vi "Calculatrice.vi"() -> ()   [LabVIEW 2020]
doc: "Calculatrice II - ceci est un programme de calculatrice"
panel:
  out "Local":string
  in  "entrée d'erreur (pas d'erreur)":errorcluster
  in  "Btn_Error":bool caption="Error"
  out "sortie d'erreur":errorcluster
  in  "Btn_Stop":bool
  out "Display":cluster{"Num":dbl, "Char":string}
  in  "Pad":T1
  # "Calculatrice"
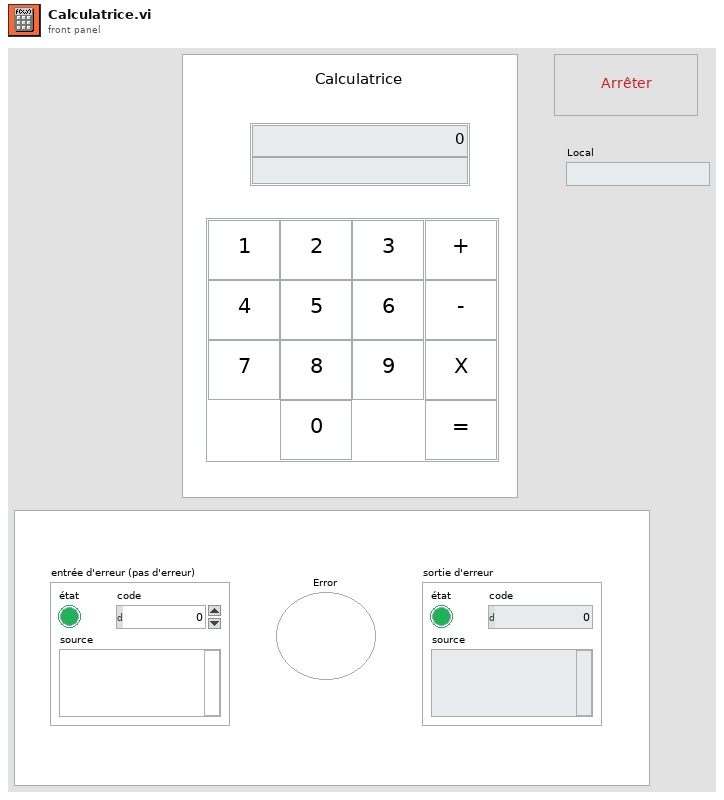
[diagram p1: front panel]
types:
  T1 = cluster{"Btn_1":bool, "Btn_2":bool, "Btn_3":bool, "Btn_4":bool, "Btn_5":bool, "Btn_6":bool, "Btn_7":bool, "Btn_8":bool, "Btn_9":bool, "Btn_0":bool, "Btn_+":bool, "Btn_-":bool, "Btn_X":bool, "Btn_=":bool}
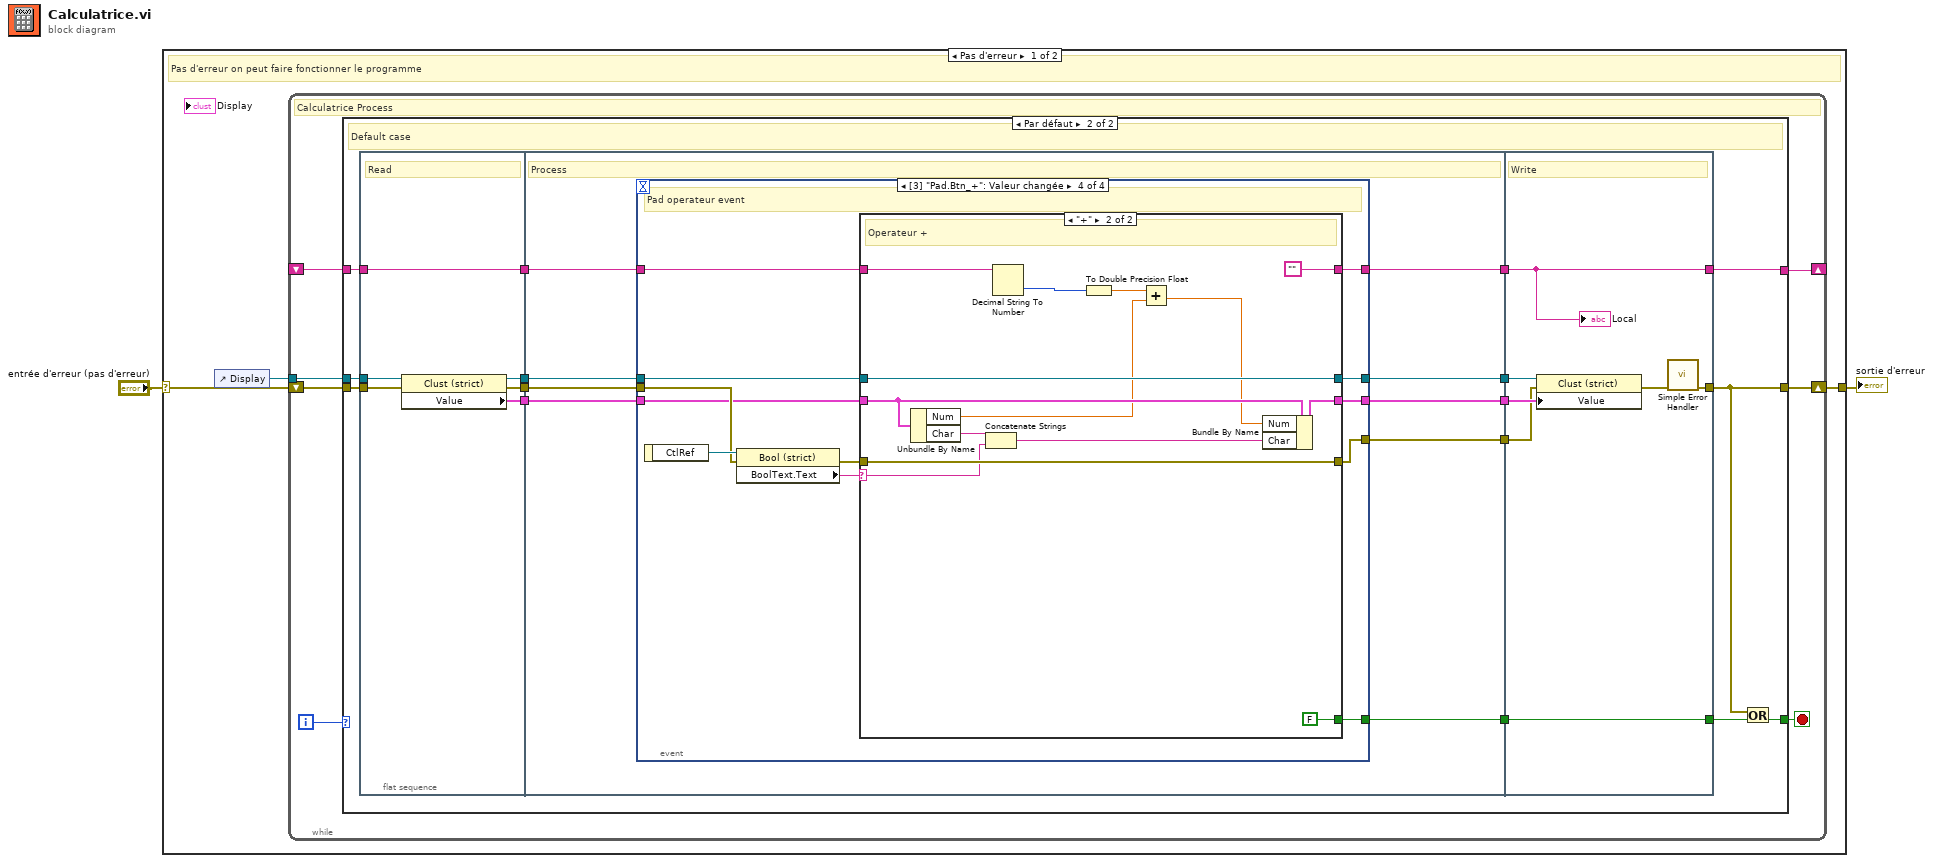
[diagram p0: block diagram]
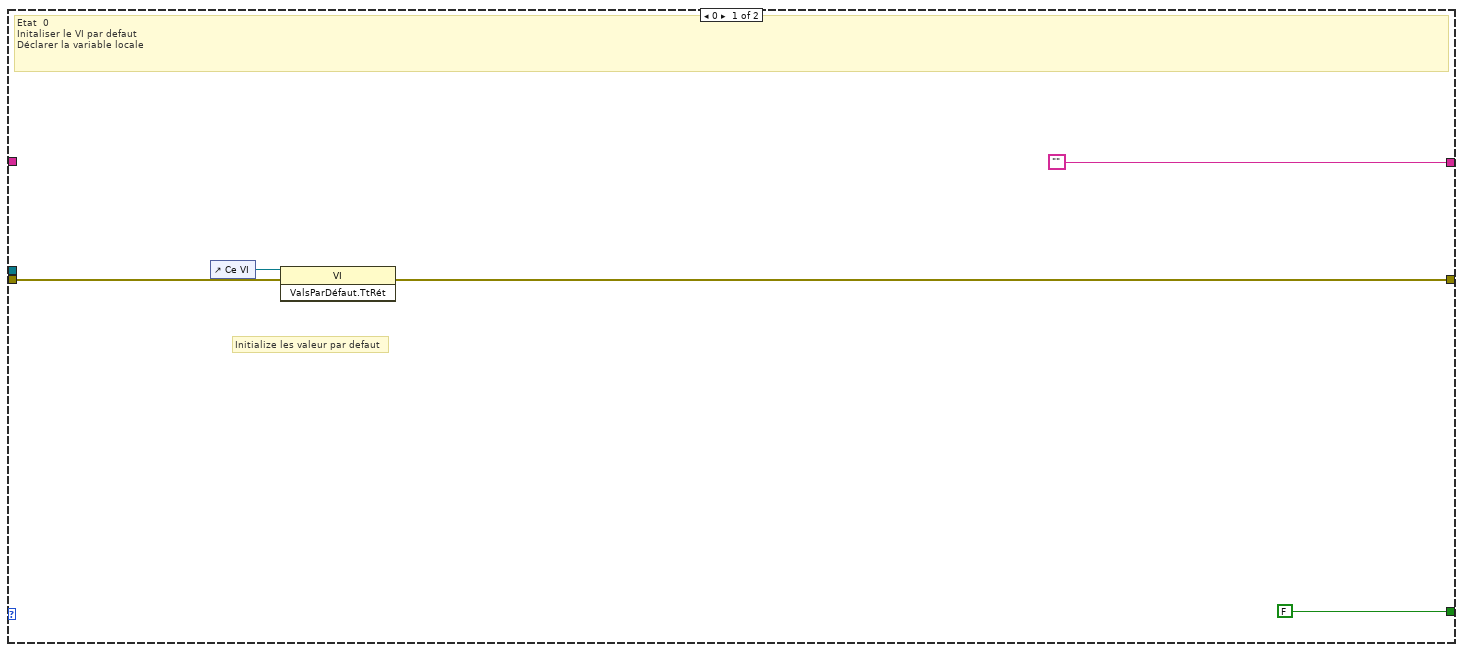
[diagram p2: hidden frame]
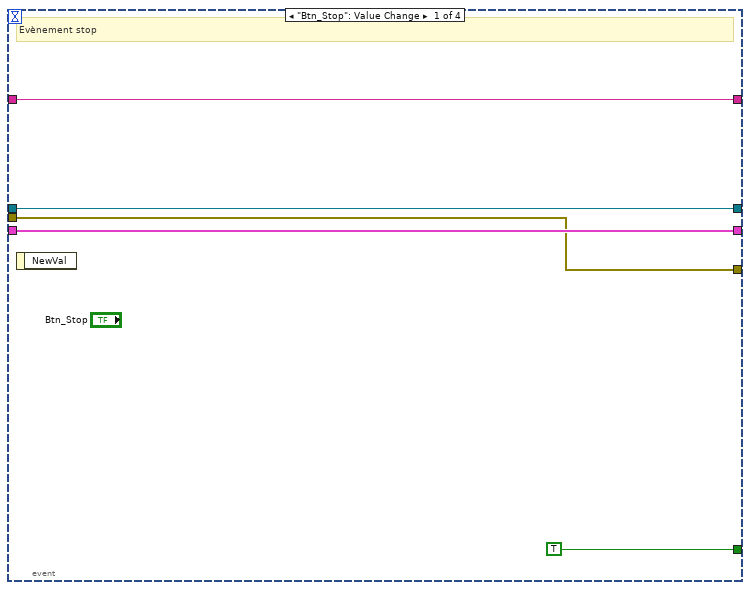
[diagram p3: hidden frame]
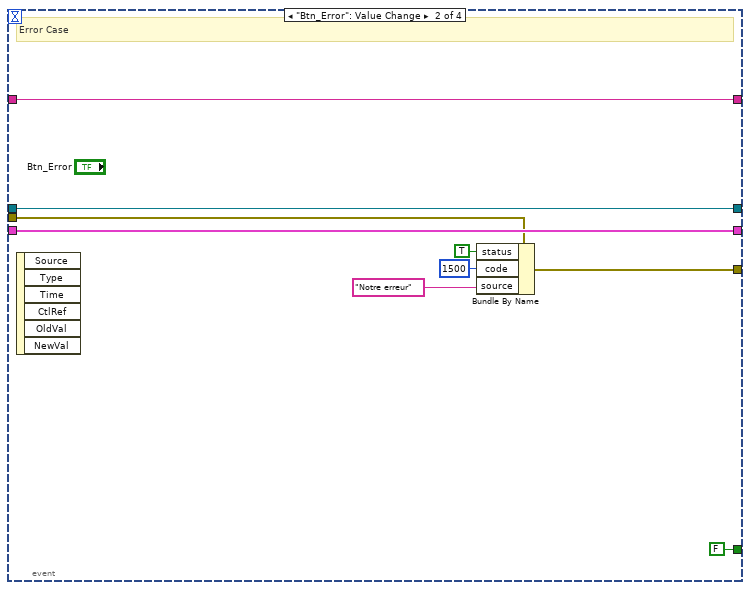
[diagram p4: hidden frame]
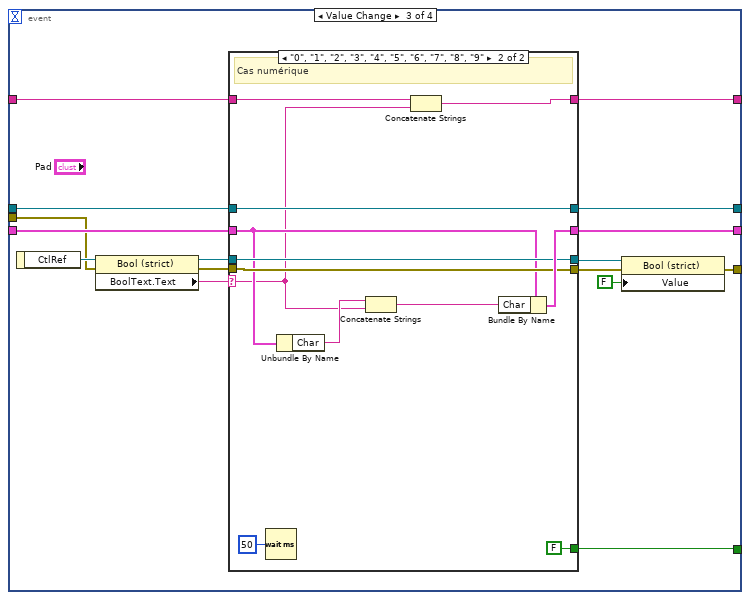
[diagram p5: hidden frame]
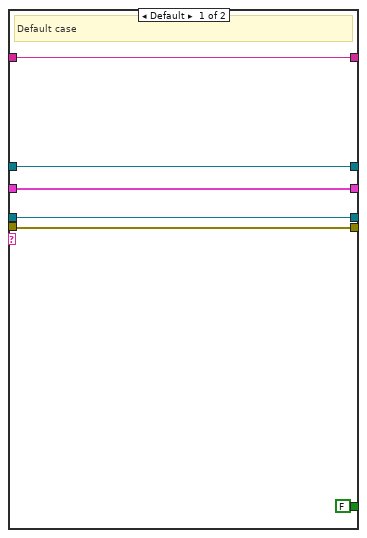
[diagram p6: hidden frame]
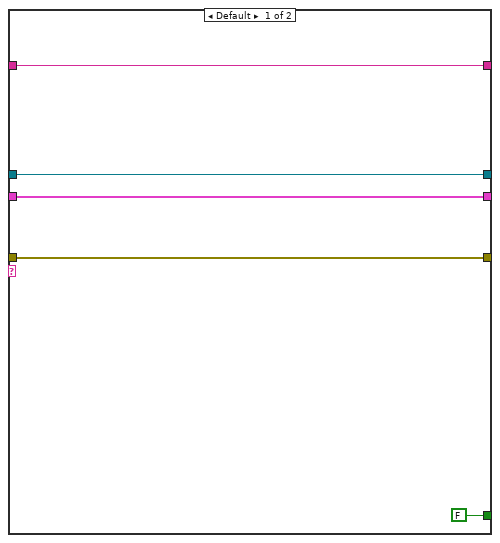
[diagram p7: hidden frame]
diagram:
  n1 = case shown="Pas d'erreur" "entrée d'erreur (pas d'erreur)" {
    selector: "entrée d'erreur (pas d'erreur)" -> [w3 w135]
    tunnel: [w4 w135] -> w2
    frame No Error {
      # "Pas d'erreur on peut faire fonctionner le programme"
      n2 = control-ref of="Display"() -> (w5:refnum<vi>)
      n3 = while {
        tunnel: w5 -> [w12]
        shift-right: [w10] -> w4
        shift-left: w3 -> [w8]
        shift-right: [w7] -> _
        shift-left: _ -> [w6]
        i -> [w9]
        stop <- w11 stop-if-true
        # "Calculatrice Process"
        n4 = case shown="Par défaut" w9 {
          tunnel: w12 -> [_ w25]
          tunnel: w8 -> [w15 w24]
          tunnel: [FALSE w23] -> w11
          tunnel: [w14 w22] -> w10
          tunnel: ["" w18] -> w7
          tunnel: w6 -> [_ w21]
          frame 0 {
            # "Initialize les valeur par defaut"
            # "Etat  0\nInitaliser le VI par defaut\nDéclarer la variable locale"
            n5 = control-ref of="Ce VI"() -> (w16:refnum<vi>)
            n6 = invoke class="VI" method="ValsParDéfaut.TtRét"(reference=w16, error in=w15) -> (error out=w14:errorcluster)  [unwired: 1 in, 2 out]
          }
          frame Default {
            # "Default case"
            n7 = flat-sequence {
              tunnel: w25 -> [w39]
              tunnel: [w38] -> w33
              tunnel: [w37] -> w32
              tunnel: w24 -> [w35]
              tunnel: [w36] -> w31
              tunnel: w21 -> [w34]
              tunnel: [w34] -> w20
              tunnel: [w48] -> w30
              tunnel: w33 -> [w47]
              tunnel: w32 -> [w46]
              tunnel: [w45] -> w29
              tunnel: [w44] -> w28
              tunnel: w31 -> [w43]
              tunnel: [w42] -> w27
              tunnel: w20 -> [w41]
              tunnel: [w40] -> w19
              tunnel: [w134] -> w26
              tunnel: w30 -> [w134]
              tunnel: w29 -> [w133]
              tunnel: w28 -> [w132]
              tunnel: w27 -> [w131]
              tunnel: [w129] -> w22
              tunnel: w19 -> [w128]
              tunnel: [w128] -> w18
              frame #0 {
                # "Read"
                n8 = property class="Clust (strict)"(reference=w39, error in=w35) -> (reference out=w37:refnum<vi>, error out=w36:errorcluster, "Value"=w38:cluster{"Num":dbl, "Char":string})
              }
              frame #1 {
                # "Process"
                n9 = event shown="[3] \"Pad.Btn_+\": Valeur changée" {
                  selector: _ -> [_ _ _ _]
                  dyn-events: _ -> [_ _ _ _]
                  timeout: _ -> [_ _ _ _]
                  tunnel: [TRUE FALSE w76 w108] -> w48
                  tunnel: w47 -> [w51 w60 w75 w104]
                  tunnel: w46 -> [w52 w61 w74 w105]
                  tunnel: [w52 w61 w73 w102] -> w45
                  tunnel: [w51 w60 w72 w103] -> w44
                  tunnel: w43 -> [w50 w59 w68 w106]
                  tunnel: [w50 w58 w65 w99] -> w42
                  tunnel: w41 -> [w49 w54 w64 w98]
                  tunnel: [w49 w54 w63 w97] -> w40
                  event "Btn_Stop": Value Change {
                    # "Evènement stop"
                    n10 = event-data() -> ()  [unwired: 1 in, 1 out]
                  }
                  event "Btn_Error": Value Change {
                    # "Error Case"
                    n11 = event-data() -> ()  [unwired: 1 in, 6 out]
                    n12 = Bundle By Name(cluster=w59, "status"=TRUE, "code"=1500, "source"="Notre erreur") -> (w58:errorcluster)
                  }
                  event "Pad.Btn_1", "Pad.Btn_2", "Pad.Btn_3", "Pad.Btn_4", "Pad.Btn_5", "Pad.Btn_6", "Pad.Btn_7", "Pad.Btn_8", "Pad.Btn_9", "Pad.Btn_0": Value Change {
                    n13 = event-data() -> ("CtlRef"=w78:refnum<vi>)  [unwired: 1 in]
                    n14 = property class="Bool (strict)"(reference=w78, error in=w68) -> (reference out=w71:refnum<vi>, error out=w67:errorcluster, "BoolText.Text"=w77:string)
                    n15 = case shown="\"0\", \"1\", \"2\", \"3\", \"4\", \"5\", \"6\", \"7\", \"8\", \"9\"" w77 {
                      selector: w77 -> [_ w85]
                      tunnel: [FALSE FALSE] -> w76
                      tunnel: w75 -> [w82 w90]
                      tunnel: w74 -> [w83 w95]
                      tunnel: [w83 w95] -> w73
                      tunnel: [w82 w94] -> w72
                      tunnel: w71 -> [w81 w93]
                      tunnel: [w81 w93] -> w70
                      tunnel: w67 -> [w80 w91]
                      tunnel: [w80 w91] -> w66
                      tunnel: w64 -> [w79 w88]
                      tunnel: [w79 w86] -> w63
                      frame Default {
                        # "Default case"
                      }
                      frame "0", "1", "2", "3", "4", "5", "6", "7", "8", "9" {
                        # "Cas numérique"
                        n16 = Wait (ms)(milliseconds to wait=u32 50 ("attente (ms)")) -> ()  [unwired: 1 out]
                        n17 = Unbundle By Name(w90) -> ("Char"=w89:string)
                        n18 = Concatenate Strings(w89, w85) -> (w87:string)
                        n19 = Concatenate Strings(w88, w85) -> (w86:string)
                        n20 = Bundle By Name(cluster=w90, "Char"=w87) -> (w94:cluster{"Num":dbl, "Char":string})
                      }
                    }
                    n21 = property class="Bool (strict)"(reference=w70, error in=w66, "Value"=FALSE ("Valeur")) -> (error out=w65:errorcluster)  [unwired: 1 out]
                  }
                  event "Pad.Btn_+": Value Change {
                    # "Pad operateur event"
                    n22 = event-data() -> ("CtlRef"=w107:refnum<vi>)  [unwired: 1 in]
                    n23 = property class="Bool (strict)"(reference=w107, error in=w106) -> (error out=w100:errorcluster, "BoolText.Text"=w101:string)  [unwired: 1 out]
                    n24 = case shown="\"+\"" w101 {
                      selector: w101 -> [_ w121]
                      tunnel: [FALSE FALSE] -> w108
                      tunnel: w105 -> [w111 w126]
                      tunnel: w104 -> [w112 w123]
                      tunnel: [w112 w124] -> w103
                      tunnel: [w111 w126] -> w102
                      tunnel: w100 -> [w110 w125]
                      tunnel: [w110 w125] -> w99
                      tunnel: w98 -> [w109 w118]
                      tunnel: [w109 ""] -> w97
                      frame Default {
                      }
                      frame "+" {
                        # "Operateur +"
                        n25 = Unbundle By Name(w123) -> ("Num"=w114:dbl, "Char"=w122:string)
                        n26 = Concatenate Strings(w122, w121) -> (w120:string)
                        n27 = Decimal String To Number(string=w118) -> (number=w117:i32)  [unwired: 2 in, 1 out]
                        n28 = To Double Precision Float(number=w117) -> (double precision float=w116:dbl)
                        n29 = Add(x=w116, y=w114) -> (x+y=w115:dbl)
                        n30 = Bundle By Name(cluster=w123, "Num"=w115, "Char"=w120) -> (w124:cluster{"Num":dbl, "Char":string})
                      }
                    }
                  }
                }
              }
              frame #2 {
                # "Write"
                n31 = property class="Clust (strict)"(reference=w133, error in=w131, "Value"=w132) -> (error out=w130:errorcluster)  [unwired: 1 out]
                n32 = call <vilib>:"Simple Error Handler.vi"("error in (no error)"=w130) -> ("error out"=w129:errorcluster)  [unwired: 4 in, 4 out]
                "Local" <- w128
              }
            }
            n33 = Or(x=w22, y=w26) -> (x .or. y?=w23:bool)
          }
        }
      }
    }
    frame Error {
      # "Erreur on n'active pas le programme"
    }
  }
  "sortie d'erreur" <- w2
